vi "(Un)Deploy SV Library.vi"(6 "Undeploy?":bool, 8 "error in (no error)":errorcluster, 11 "Library path":path) -> (0 "error out":errorcluster)   [LabVIEW 2026, in "TALOS.lvlib" / "Classes.lvlib" / "Circus Shared Variables.lvclass"]
doc: "This VI is used to (un)deploy a library of SVs."
uses:
  Circus Shared Variables.lvclass
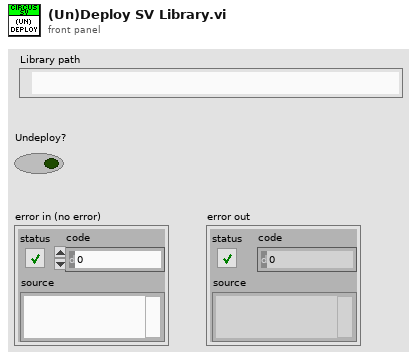
[diagram p1: front panel]
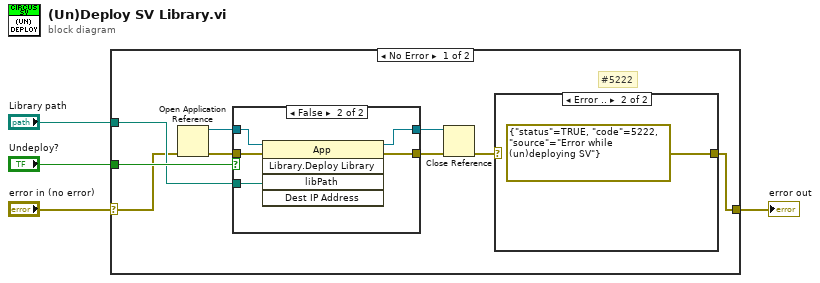
[diagram p0: block diagram]
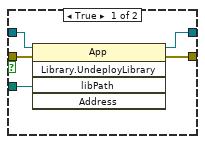
[diagram p3: hidden frame]
diagram:
  n1 = case shown="No Error" "error in (no error)" {
    selector: "error in (no error)" -> [w11 w26]
    tunnel: "Undeploy?" -> [w13 _]
    tunnel: [w5 w26] -> w3
    tunnel: "Library path" -> [w12 _]
    frame No Error {
      # "#5222"
      n2 = Open Application Reference(8:w11) -> (0:w9:errorcluster, 3:w10:refnum<vi>)  [unwired: 3 in]
      n3 = case shown="False" w13 {
        tunnel: w10 -> [w20 w25]
        tunnel: w9 -> [w19 w24]
        tunnel: [w18 w23] -> w8
        tunnel: [w17 w22] -> w7
        tunnel: w12 -> [w16 w21]
        frame True {
          n4 = invoke class="App" method="Library.UndeployLibrary"(reference=w20, error in=w19, "libPath"=w16) -> (reference out=w17:refnum<vi>, error out=w18:errorcluster)  [unwired: 2 in, 3 out]
        }
        frame False {
          n5 = invoke class="App" method="Library.Deploy Library"(reference=w25, error in=w24, "libPath"=w21) -> (reference out=w22:refnum<vi>, error out=w23:errorcluster)  [unwired: 2 in, 3 out]
        }
      }
      n6 = Close Reference(reference=w7, error in (no error)=w8) -> (error out=w6:errorcluster)
      n7 = case shown="Error .." w6 {
        selector: w6 -> [w14 _]
        tunnel: [w14 errorcluster {"status"=TRUE, "code"=5222, "source"="Error while (un)deploying SV"} ("error IO")] -> w5
        frame No Error {
        }
        frame Error {
        }
      }
    }
    frame Error {
    }
  }
  "error out" <- w3
